vi "test_GPIB to RS-xxx ConvBox Read.vi"(8 "error in (no error)":errorcluster, 11 "TestCase in":refnum<class "Serial Protocols Tests.lvclass">) -> (0 "error out":errorcluster, 3 "TestCase out":refnum<class "Serial Protocols Tests.lvclass">)   [LabVIEW 2019, in "Serial Protocols Tests.lvclass"]
uses:
  Serial Protocols Tests.lvclass
  Listener/Listener.lvclass
  Listener/ListenerClassControls/Operation.ctl
  RS-xxx to GPIB ConvBox/RS-xxx to GPIB ConvBox.lvclass
  D:/GitRepository/niveristand-instrument-addon-classes/Source/Protocols/Protocol Parent/Protocol Parent.lvclass
  <vilib>/Platform/TimedLoop/XDataNode/timing_clust.ctl
  <vilib>/Platform/TimedLoop/XDataNode/nitl_modes.ctl
  <vilib>/Platform/TimedLoop/XDataNode/wakeup.ctl
  RS-xxx to GPIB ConvBox/RS-xxx to GPIB ConvBox.lvclass/RS-xxx to GPIB ConvBox.ctl
  Protocol Parent/Methods/Read Parameter.ctl
  RS-xxx to GPIB ConvBox/Data Access/Write GPIB Address.vi
  59c794b9-68da-454b-bfb7-ac37d142d7af.vi
  RS-xxx to GPIB ConvBox/Data Access/Write ConvBox Address.vi
  RS-xxx to GPIB ConvBox/Data Access/Write Port.vi
  <vilib>/platform/TimedLoop/XDataNode/XDataNode.xnode
  <vilib>/addons/_JKI Toolkits/VI Tester/TestCase.llb/TestCase.lvclass
  <vilib>/Platform/TimedLoop/XDataNode/XDNodeRunTimeDep.lvlib
  Protocol Parent/Protocol Parent.lvclass
  C:/Program Files (x86)/National Instruments/LabVIEW 2019/vi.lib/addons/_JKI Toolkits/VI Tester/TestCase.llb/TestCase.lvclass
panel:
  out "Array":string[](array[string])
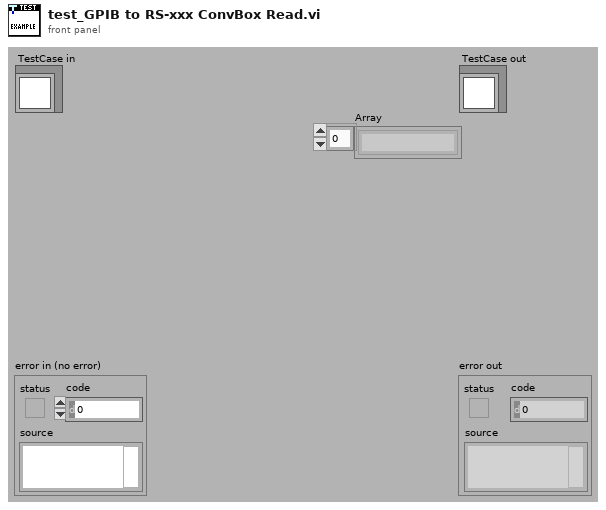
[diagram p1: front panel]
types:
  T1 = typedef "Listener.lvclass/Operation.ctl" = enum16{"Read", "Write"}
  T2 = typedef "XDNodeRunTimeDep.lvlib/timing_clust.ctl" = cluster{"Expected End [f-1]":u64, "Actual End [f-1]":u64, "Finished Late? [f-1]":bool, "Expected End [i-1]":u64, "Actual End [i-1]":u64, "Finished Late? [i-1]":bool, "Expected Start [i]":u64, "Actual Start [i]":u64, "Expected Start [f]":u64, "Actual Start [f]":u64, "Source Name":string, "Structure Name":string, "Period":i64, "Deadline":i64, "Offset":i64, "Start":i64, "Priority":i32, "Timeout":i32, "Mode":T3, "Wakeup Reason":T4, "Error":errorcluster, "Source Type":string, "Secondary Source Type":string, "Global End Time":u64, "Global Start Time":u64, "Frame Duration":u64, "Iteration Duration":u64, "Assigned CPU":i32, "I/O Scan Engine Mode":u32}
  T3 = typedef "XDNodeRunTimeDep.lvlib/nitl_modes.ctl" = enum32{"No Change", "Process missed periods, maintain original phase", "Discard missed periods, maintain original phase", "Process missed periods, ignore original phase", "Discard missed periods, ignore original phase"}
  T4 = typedef "XDNodeRunTimeDep.lvlib/wakeup.ctl" = enum32{"Normal", "Aborted", "Asynchronous wakeup", "Timing source error", "Timed loop error", "Timeout"}
  T5 = typedef "Protocols.lvlib/Protocol Parent.lvclass/Read Parameter.ctl" = cluster{"Wait Type":enum16{"Byte Count", "Wait sec"}, "Wait Value":dbl}
  T6 = typedef "Listener.lvclass/RS-xxx To GPIB ConvBox Data Structure.ctl" = cluster{"Protocol Port Ref":refnum<visa-resource-name>, "Listener Port Ref":refnum<visa-resource-name>, "Data":string, "Command Messages Read":string[], "Address":string}
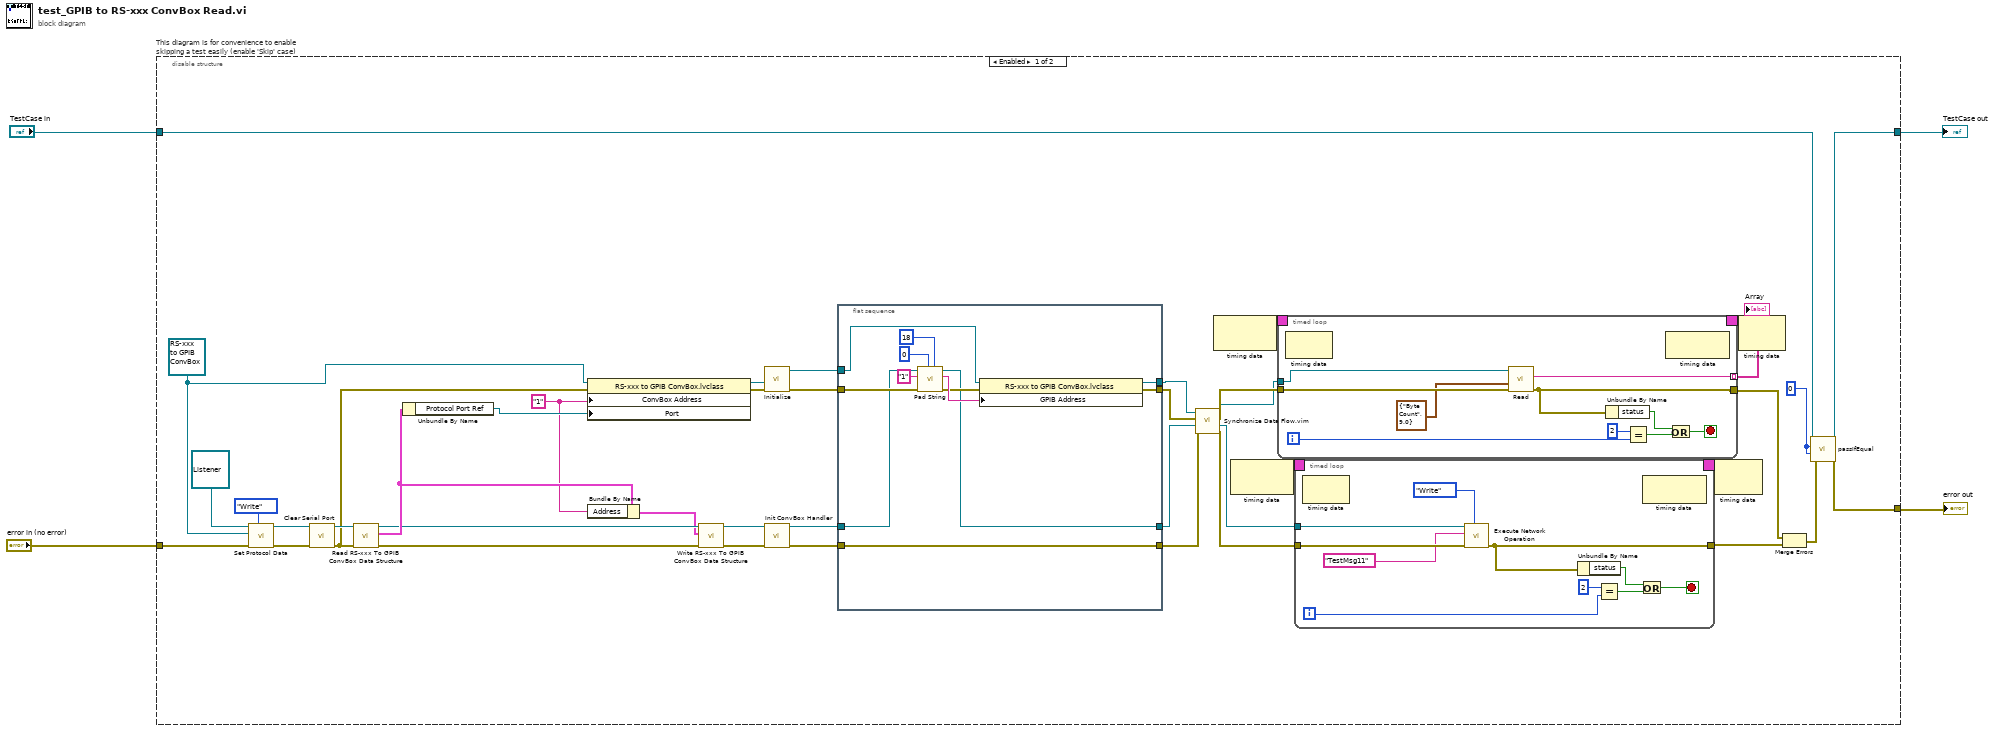
[diagram p0: block diagram]
diagram:
  n1 = disable-structure "This diagram is for convenience to enable skipping a test easily (enable 'Skip' case)" shown="Enabled" {
    disable-tunnel: "TestCase in" -> [w46 w90]
    disable-tunnel: [w38 w88] -> w1
    disable-tunnel: [w39 w89] -> w3
    disable-tunnel: "error in (no error)" -> [w43 w87]
    frame Enabled {
      w21 = 0
      w11 = "1" ("ConvBox Address")
      w35 = refnum<class "RS-xxx to GPIB ConvBox.lvclass"> refnum ("Protocols.lvlib:RS-xxx to GPIB ConvBox.lvclass")
      n2 = call "Set Protocol Data.vi"("Operation"=Operation."Write", "error in (no error)"=w43, "Protocols.lvlib:Protocol Parent.lvclass"=w35, "Listener In.lvclass"=refnum<class "Listener.lvclass"> refnum ("Listener.lvclass")) -> ("error out"=w42:errorcluster, "Listener Out.lvclass"=w41:refnum<class "Listener.lvclass">)  [unwired: 6 in]
      n3 = call "Clear Serial Port.vi"("error in (no error)"=w42, "Listener In.lvclass"=w41) -> ("error out"=w36:errorcluster, "Listener out"=w40:refnum<class "Listener.lvclass">)  [unwired: 8 in]
      n4 = call-dynamic "Read RS-xxx To GPIB ConvBox Data Structure.vi"("error in (no error)"=w36, "Listener in"=w40) -> ("error out"=w10:errorcluster, "RS-xxx To GPIB ConvBox Data Structure"=w12:T6, "Listener out"=w7:refnum<class "Listener.lvclass">)  [unwired: 7 in]
      n5 = Unbundle By Name(w12) -> ("Protocol Port Ref"=w37:refnum<visa-resource-name>)
      n6 = property class="RS-xxx to GPIB ConvBox.lvclass"(reference=w35, error in=w36, "ConvBox Address"=w11, "Port"=w37) -> (reference out=w33:refnum<class "RS-xxx to GPIB ConvBox.lvclass">, error out=w34:errorcluster)
      n7 = Bundle By Name(cluster=w12, "Address"=w11) -> (w6:T6)
      n8 = call-dynamic "Write RS-xxx To GPIB ConvBox Data Structure.vi"("error in (no error)"=w10, "RS-xxx To GPIB ConvBox Data Structure"=w6, "Listener in"=w7) -> ("error out"=w9:errorcluster, "Listener out"=w8:refnum<class "Listener.lvclass">)  [unwired: 7 in]
      n9 = call-dynamic "Initialize.vi"("error in (no error)"=w34, "RS232 to GPIB ConvBox in"=w33) -> ("error out"=w32:errorcluster, "RS232 to GPIB ConvBox out"=w29:refnum<class "RS-xxx to GPIB ConvBox.lvclass">)  [unwired: 8 in]
      n10 = call "Init ConvBox Handler.vi"("error in (no error)"=w9, "Listener in"=w8) -> ("error out"=w31:errorcluster, "Listener out"=w30:refnum<class "Listener.lvclass">)  [unwired: 8 in]
      n11 = flat-sequence {
        tunnel: w32 -> [w86]
        tunnel: w31 -> [w79]
        tunnel: w30 -> [w76]
        tunnel: w29 -> [w80]
        tunnel: [w79] -> w17
        tunnel: [w75] -> w18
        tunnel: [w78] -> w19
        tunnel: [w77] -> w20
        frame #0 {
          n12 = call "Pad String.vi"("Expected Length"=u8 18, "Pad Character"=u8 0, "error in (no error)"=w86, "String To Pad"="1", "Listener in"=w76) -> ("error out"=w81:errorcluster, "Padded String"=w82:string, "Listener out"=w75:refnum<class "Listener.lvclass">)  [unwired: 4 in]
          n13 = property class="RS-xxx to GPIB ConvBox.lvclass"(reference=w80, error in=w81, "GPIB Address"=w82) -> (reference out=w77:refnum<class "RS-xxx to GPIB ConvBox.lvclass">, error out=w78:errorcluster)
        }
      }
      n14 = call "Synchronize Data Flow.vim"("input 4"=w17, "input 3"=w18, "input 2"=w19, "input 1"=w20) -> ("output 4"=w16:errorcluster, "output 3"=w15:refnum<class "Listener.lvclass">, "output 2"=w14:errorcluster, "output 1"=w13:refnum<class "RS-xxx to GPIB ConvBox.lvclass">)
      n15 = node-c288() -> (w28:T2)  [unwired: 1 in]
      n16 = node-c288() -> (w26:T2)  [unwired: 1 in]
      n17 = timed-loop {
        timing: w28 -> [_]
        timing-out: [_] -> w27
        tunnel: w13 -> [w69]
        tunnel: w14 -> [w70]
        tunnel: [w62] -> w24
        tunnel: [w61] -> w5 mode=indexing
        i -> [w66]
        stop <- w63 stop-if-true
        n18 = node-c288() -> ()  [unwired: 1 in, 1 out]
        n19 = call-dynamic "Read.vi"("error in (no error)"=w70, "Variant"=T5 {"Wait Type"=enum."Byte Count", "Wait Value"=9.0} ("Read Parameter"), "RS232 to GPIB ConvBox in"=w69) -> ("error out"=w62:errorcluster, "String"=w61:string)  [unwired: 6 in, 1 out]
        n20 = Unbundle By Name(w62) -> ("status"=w67:bool)
        n21 = Equal?(x=2, y=w66) -> (x = y?=w64:bool)
        n22 = node-c288() -> ()  [unwired: 1 in, 1 out]
        n23 = Or(x=w67, y=w64) -> (x .or. y?=w63:bool)
      }
      "Array" <- w5
      n24 = timed-loop {
        timing: w26 -> [_]
        timing-out: [_] -> w25
        tunnel: w16 -> [w56]
        tunnel: w15 -> [w55]
        tunnel: [w50] -> w23
        i -> [w47]
        stop <- w49 stop-if-true
        n25 = node-c288() -> ()  [unwired: 1 in, 1 out]
        n26 = call "Execute Network Operation.vi"("Operation"=Operation."Write", "error in (no error)"=w56, "Message"="TestMsg11", "Listener In.lvclass"=w55) -> ("error out"=w50:errorcluster)  [unwired: 6 in, 1 out]
        n27 = Unbundle By Name(w50) -> ("status"=w51:bool)
        n28 = Equal?(x=2, y=w47) -> (x = y?=w53:bool)
        n29 = Or(x=w51, y=w53) -> (x .or. y?=w49:bool)
        n30 = node-c288() -> ()  [unwired: 1 in, 1 out]
      }
      n31 = node-c288(w25) -> ()  [unwired: 1 out]
      n32 = node-c288(w27) -> ()  [unwired: 1 out]
      n33 = Merge Errors(w24, w23) -> (w22:errorcluster)
      n34 = call-dynamic "passIfEqual.vi"("error in (no error)"=w22, "y"=w21, "x"=w21, "TestCase in"=w46) -> ("error out"=w39:errorcluster, "TestCase out"=w38:refnum<class "Serial Protocols Tests.lvclass">)  [unwired: 6 in]
    }
    frame Disabled {
      # "skip test result while test is under development"
      n35 = call <vilib>:"skip.vi"("error in (no error)"=w87, "TestCase in"=w90) -> ("error out"=w89:errorcluster, "TestCase out"=w88:refnum<class "Serial Protocols Tests.lvclass">)  [unwired: 8 in]
    }
  }
  "error out" <- w3
  "TestCase out" <- w1
